vi "APS spiral ca.vi"(0 "Axis_ID_Array":i32, 1 "Option":i32, 2 "CenterArray":dbl, 3 "NormalArray":dbl, 4 "Angle":dbl, 5 "DeltaH":dbl, 6 "FinalR":dbl, 7 "error in (no error)":errorcluster caption="错误输入（无错误）", 8 "TransPara":dbl, 9 "Wait":cluster{"h_event":u32, "i32_ret":i32}) -> (18 "TransPara out":dbl, 19 "Wait out":cluster{"h_event":u32, "i32_ret":i32}, 20 "Axis_ID_Array out":i32, 21 "function return":i32, 22 "CenterArray out":dbl, 23 "NormalArray out":dbl, 27 "error out":errorcluster caption="错误输出")   [LabVIEW 2011, in "APS168.lvlib"]
doc: "I32 FNTYPE APS_spiral_ca( I32 *Axis_ID_Array, I32 Option, F64 *CenterArray, F64 *NormalArray, F64 Angle, F64 DeltaH, F64 FinalR, F64 *TransPara, ASYNCALL *Wait );"
uses:
  APS168.lvlib
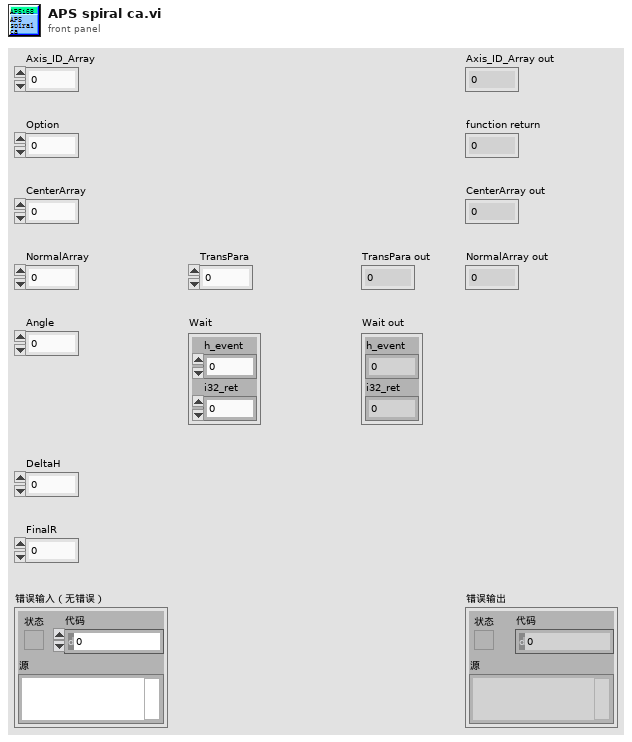
[diagram p1: front panel]
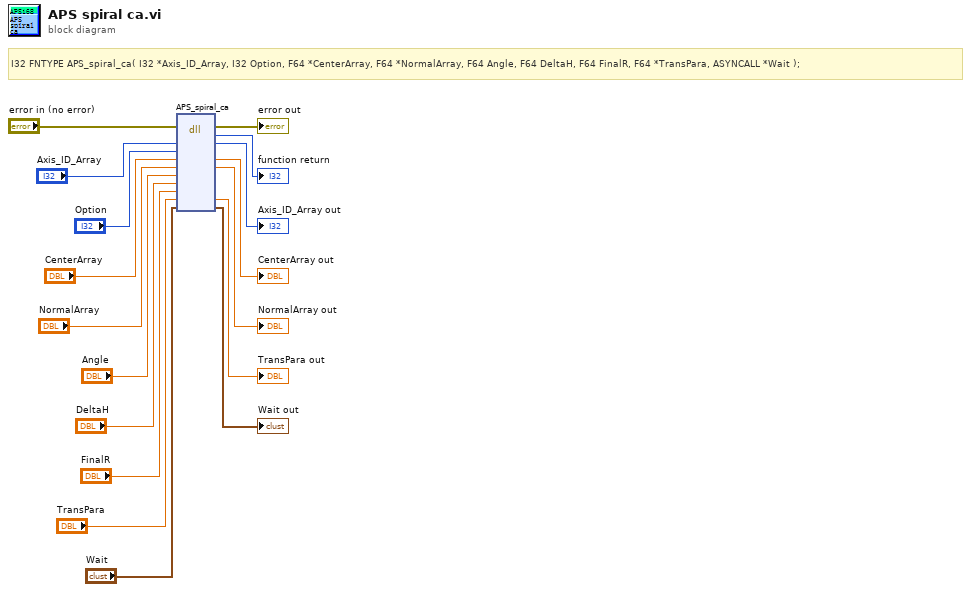
[diagram p0: block diagram]
diagram:
  # "I32 FNTYPE APS_spiral_ca( I32 *Axis_ID_Array, I32 Option, F64 *CenterArray, F64 *NormalArray, F64 Angle, F64 DeltaH, F64 FinalR, F64 *TransPara, ASYNCALL *Wait );"
  n1 = dll-call lib="PTH1Labs E软件ADLINK 204CAPS_1_7_1_LIB line 连续运动204APS168.*" fn="APS_spiral_ca"(error in="error in (no error)", "Axis_ID_Array"="Axis_ID_Array", "Option"="Option", "CenterArray"="CenterArray", "NormalArray"="NormalArray", "Angle"="Angle", "DeltaH"="DeltaH", "FinalR"="FinalR", "TransPara"="TransPara", "Wait"="Wait") -> (error out=→"error out":errorcluster, →"function return":i32, "Axis_ID_Array"=→"Axis_ID_Array out":i32, "CenterArray"=→"CenterArray out":dbl, "NormalArray"=→"NormalArray out":dbl, "TransPara"=→"TransPara out":dbl, "Wait"=→"Wait out":cluster{"h_event":u32, "i32_ret":i32})  [unwired: 6 in, 1 out]
